vi "Help VI.vi"() -> ()   [LabVIEW 2016]
panel:
  out "String":string
  in  "stop":bool
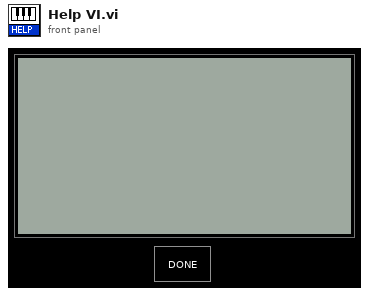
[diagram p1: front panel]
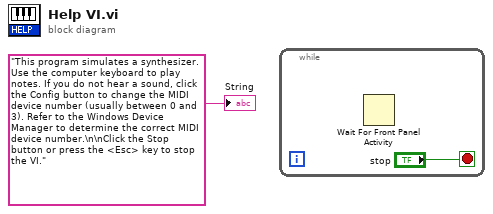
[diagram p0: block diagram]
diagram:
  n1 = while {
    stop <- "stop" stop-if-true
    n2 = Wait For Front Panel Activity() -> ()  [unwired: 3 in, 1 out]
  }
  "String" <- "This program simulates a synthesizer. Use the computer keyboard to play notes. If you do not hear a sound, click the Config button to change the MIDI device number (usually between 0 and 3). Refer to the Windows Device Manager to determine the correct MIDI device number.\n\nClick the Stop button or press the <Esc> key to stop the VI." ("String")
